vi "Startup_FGGA_selection.vi"(0 "VISA resource name":refnum<visa-resource-name>="ASRL7::INSTR") -> (4 "VISA resource name out":refnum<visa-resource-name>, 8 "old FGGA = True\nnew FGGA = False":bool, 15 "error out":errorcluster)   [LabVIEW 2014]
uses:
  <vilib>/Platform/TimedLoop/XDataNode/timing_clust.ctl
  <vilib>/Platform/TimedLoop/XDataNode/nitl_modes.ctl
  <vilib>/Platform/TimedLoop/XDataNode/wakeup.ctl
  <vilib>/Instr/_visa.llb/VISA Set IO Buffer Mask.ctl
  <vilib>/Instr/_visa.llb/VISA Flush IO Buffer Mask.ctl
  <vilib>/Instr/_visa.llb/VISA Configure Serial Port (Instr).vi
  <vilib>/platform/TimedLoop/XDataNode/XDataNode.xnode
  <vilib>/Platform/TimedLoop/XDataNode/XDNodeRunTimeDep.lvlib
panel:
  in  "New FGGA timeout":u32=10000
  in  "Old FGGA timeout":u32=2000
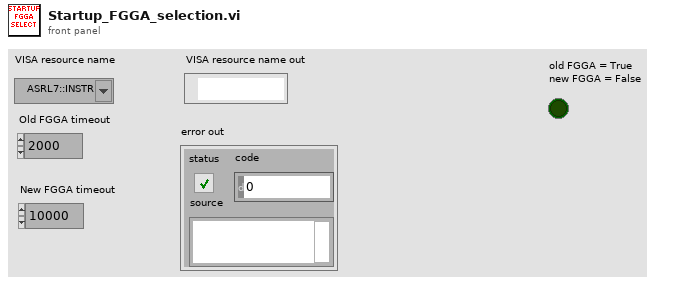
[diagram p1: front panel]
types:
  T1 = typedef "XDNodeRunTimeDep.lvlib/timing_clust.ctl" = cluster{"Expected End [f-1]":u64, "Actual End [f-1]":u64, "Finished Late? [f-1]":bool, "Expected End [i-1]":u64, "Actual End [i-1]":u64, "Finished Late? [i-1]":bool, "Expected Start [i]":u64, "Actual Start [i]":u64, "Expected Start [f]":u64, "Actual Start [f]":u64, "Source Name":string, "Structure Name":string, "Period":i64, "Deadline":i64, "Offset":i64, "Start":i64, "Priority":i32, "Timeout":i32, "Mode":T2, "Wakeup Reason":T3, "Error":errorcluster, "Source Type":string, "Secondary Source Type":string, "Global End Time":u64, "Global Start Time":u64, "Frame Duration":u64, "Iteration Duration":u64, "Assigned CPU":i32, "I/O Scan Engine Mode":u32}
  T2 = typedef "XDNodeRunTimeDep.lvlib/nitl_modes.ctl" = enum32{"No Change", "Process missed periods, maintain original phase", "Discard missed periods, maintain original phase", "Process missed periods, ignore original phase", "Discard missed periods, ignore original phase"}
  T3 = typedef "XDNodeRunTimeDep.lvlib/wakeup.ctl" = enum32{"Normal", "Aborted", "Asynchronous wakeup", "Timing source error", "Timed loop error", "Timeout"}
  T4 = typedef "VISA Flush IO Buffer Mask.ctl" = u16
  T5 = typedef "VISA Set IO Buffer Mask.ctl" = u16
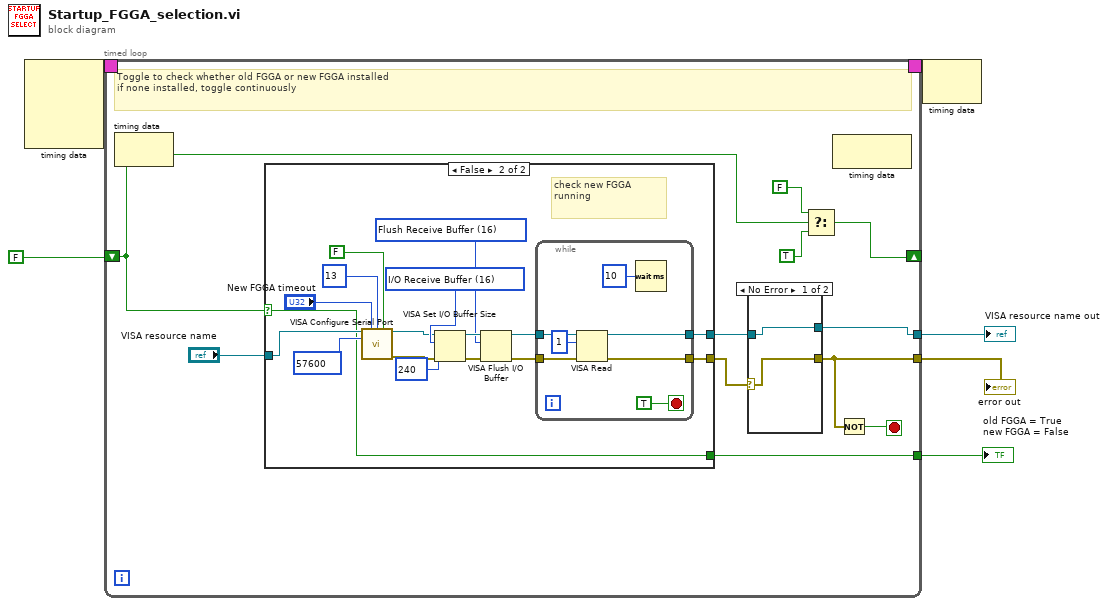
[diagram p0: block diagram]
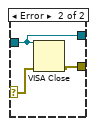
[diagram p2: hidden frame]
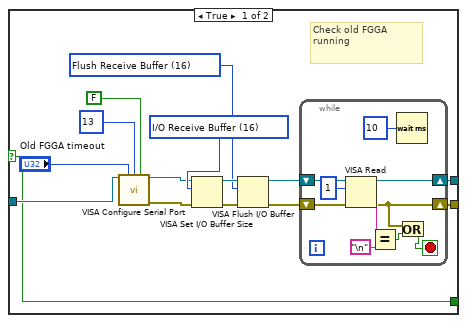
[diagram p3: hidden frame]
diagram:
  n1 = node-c288() -> (w3:T1)  [unwired: 4 in]
  n2 = timed-loop {
    tunnel: [w12] -> w4
    tunnel: [w10] -> w5
    shift-right: [w14] -> _
    shift-left: FALSE -> [w8]
    timing: w3 -> [_]
    timing-out: [_] -> w2
    tunnel: [w7] -> w1
    stop <- w17 stop-if-true
    # "Toggle to check whether old FGGA or new FGGA installed\nif none installed, toggle continuously"
    n3 = node-c288() -> ()  [unwired: 1 in, 1 out]
    n4 = case shown="False" w8 {
      selector: w8 -> [w36 w52]
      tunnel: [w39 w56] -> w13
      tunnel: [w38 w55] -> w11
      tunnel: "VISA resource name" -> [w37 w53]
      tunnel: [w36 w52] -> w7
      frame True {
        w30 = T4 16 items=["Flush Receive Buffer"=16, "Write Transmit Buffer to Device"=32, "Flush Receive Buffer (No I/O)"=64, "Flush Transmit Buffer"=128] ("Mask")
        w31 = T5 16 items=["I/O Receive Buffer"=16, "I/O Transmit Buffer"=32, "I/O Receive and Transmit Buffer"=48] ("Mask")
        # "Check old FGGA\nrunning"
        n5 = call-poly "VISA Configure Serial Port"("VISA resource name"=w37, "timeout (10sec)"="Old FGGA timeout", "termination char\n(0xA = '\\n' = LF)"=u8 13 ("termination char\n(0xA = '\\n' = LF)"), "Enable Termination\nChar (T)"=FALSE ("Enable Termination\nChar (T)")) -> ("VISA resource name out"=w29:refnum<visa-resource-name>, "error out"=w28:errorcluster)  [unwired: 10 in]
        n6 = VISA Set I/O Buffer Size(VISA resource name=w29, mask (16)=w31, error in (no error)=w28) -> (VISA resource name out=w32:refnum<visa-resource-name>, error out=w33:errorcluster)  [unwired: 1 in]
        n7 = VISA Flush I/O Buffer(VISA resource name=w32, mask (16)=w30, error in (no error)=w33) -> (VISA resource name out=w27:refnum<visa-resource-name>, error out=w26:errorcluster)
        n8 = while {
          shift-right: [w47] -> w38
          shift-left: w27 -> [w49]
          shift-right: [w41] -> w39
          shift-left: w26 -> [w48]
          stop <- w42 stop-if-true
          n9 = VISA Read(VISA resource name=w49, byte count=u32 1, error in (no error)=w48) -> (VISA resource name out=w47:refnum<visa-resource-name>, read buffer=w43:string, error out=w41:errorcluster)  [unwired: 1 out]
          n10 = Equal?(x=w43, y="\n") -> (x = y?=w44:bool)
          n11 = Wait (ms)(milliseconds to wait=u32 10) -> ()  [unwired: 1 out]
          n12 = Or(x=w41, y=w44) -> (x .or. y?=w42:bool)
        }
      }
      frame False {
        w61 = T4 16 items=["Flush Receive Buffer"=16, "Write Transmit Buffer to Device"=32, "Flush Receive Buffer (No I/O)"=64, "Flush Transmit Buffer"=128] ("Mask")
        w62 = T5 16 items=["I/O Receive Buffer"=16, "I/O Transmit Buffer"=32, "I/O Receive and Transmit Buffer"=48] ("Mask")
        # "check new FGGA\nrunning"
        n13 = call-poly "VISA Configure Serial Port"("VISA resource name"=w53, "timeout (10sec)"="New FGGA timeout", "termination char\n(0xA = '\\n' = LF)"=u8 13 ("termination char\n(0xA = '\\n' = LF)"), "Enable Termination\nChar (T)"=FALSE ("Enable Termination\nChar (T)"), "baud rate (9600)"=u32 57600) -> ("VISA resource name out"=w60:refnum<visa-resource-name>, "error out"=w59:errorcluster)  [unwired: 9 in]
        n14 = VISA Set I/O Buffer Size(VISA resource name=w60, mask (16)=w62, size (4096)=u32 240, error in (no error)=w59) -> (VISA resource name out=w63:refnum<visa-resource-name>, error out=w64:errorcluster)
        n15 = VISA Flush I/O Buffer(VISA resource name=w63, mask (16)=w61, error in (no error)=w64) -> (VISA resource name out=w58:refnum<visa-resource-name>, error out=w57:errorcluster)
        n16 = while {
          tunnel: w57 -> [w72]
          tunnel: [w69] -> w56
          tunnel: w58 -> [w73]
          tunnel: [w71] -> w55
          stop <- TRUE stop-if-true
          n17 = VISA Read(VISA resource name=w73, byte count=u32 1, error in (no error)=w72) -> (VISA resource name out=w71:refnum<visa-resource-name>, error out=w69:errorcluster)  [unwired: 2 out]
          n18 = Wait (ms)(milliseconds to wait=u32 10) -> ()  [unwired: 1 out]
        }
      }
    }
    n19 = case shown="No Error" w13 {
      selector: w13 -> [w20 w24]
      tunnel: [w20 w23] -> w12
      tunnel: w11 -> [w21 w22]
      tunnel: [w21 w22] -> w10
      frame No Error {
      }
      frame Error {
        n20 = VISA Close(VISA resource name=w22, error in (no error)=w24) -> (error out=w23:errorcluster)
      }
    }
    n21 = Select(t=FALSE, s=w8, f=TRUE) -> (s? t:f=w14:bool)
    n22 = node-c288() -> ()  [unwired: 1 in, 1 out]
    n23 = Not(x=w12) -> (.not. x?=w17:bool)
  }
  "VISA resource name out" <- w5
  "error out" <- w4
  "old FGGA = True\nnew FGGA = False" <- w1
  n24 = node-c288(w2) -> ()  [unwired: 1 out]
